vi "SENS_CORR_EXT_AUTO_LOSS.vi"(0 "VISA IN":refnum<visa-resource-name>, 1 "Include Loss Correction ON/OFF":bool, 5 "error in":errorcluster, 7 "Channel":i32) -> (14 "VISA Out":refnum<visa-resource-name>, 19 "error out":errorcluster)   [LabVIEW 2018, in "PNA-X.lvlib"]
doc: "SENSe<cnum>:CORRection:EXTension:AUTO:LOSS <bool> \n(Read-Write) Specifies whether or not to include loss correction as part of automatic port extension. \nLearn more about Loss Compensation in port extension. \nParameters \n<cnum> Any existing channel number. If unspecified, value is set to 1 \n<bool> ON (or 1) - Includes Loss correction. \nOFF (or 0) - Does NOT include Loss correction. \nExamples SENS:CORR:EXT:AUTO:LOSS 1 \nsense2:correction:extension:auto:loss off \nQuery Syntax SENSe<cnum>:CORRection:EXTension:AUTO:LOSS? \nReturn Type Boolean \nDefault OFF (0)"
uses:
  PNA-X.lvlib
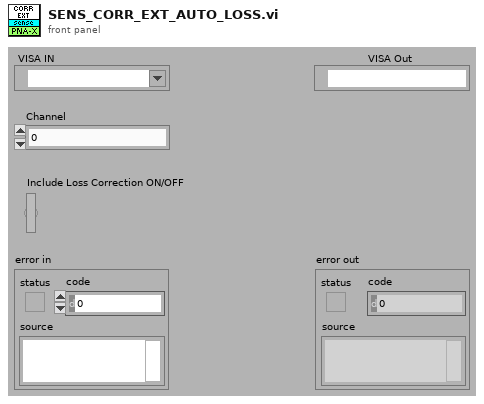
[diagram p1: front panel]
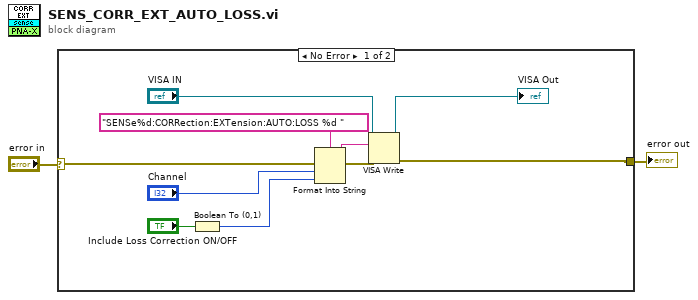
[diagram p0: block diagram]
diagram:
  n1 = case shown="No Error" "error in" {
    selector: "error in" -> [w12 w13]
    tunnel: [w7 w13] -> w1
    frame No Error {
      n2 = Boolean To (0,1)(Boolean="Include Loss Correction ON/OFF") -> (0, 1=w3:i16)
      n3 = Format Into String(format string="SENSe%d:CORRection:EXTension:AUTO:LOSS %d " ("Cmdline"), error in=w12, "Channel", w3) -> (resulting string=w10:string, error out=w11:errorcluster)  [unwired: 1 in]
      n4 = VISA Write(VISA resource name="VISA IN", write buffer=w10, error in (no error)=w11) -> (VISA resource name out=→"VISA Out":refnum<visa-resource-name>, error out=w7:errorcluster)  [unwired: 1 out]
    }
    frame Error {
    }
  }
  "error out" <- w1
